vi "mlink_scan_trigger_encoder.vi"(6 "module":u8, 7 "trigger type":T1, 8 "error in (no error)":errorcluster, 9 "slope":u8, 10 "position":i32, 11 "connection ID":i32=-1) -> (0 "error out":errorcluster, 3 "connection ID out":i32)   [LabVIEW 2009, in "MicroDAQ.lvlib" / "mlink.lvlib"]
doc: "This function configures Encoder value trigger for AO/AI scan operation. The function shall \nbe called after scan initialization function. The trigger argument determines if function affects \nAO or AI trigger settings. The module argument determines which encoder module position \nvalue will be used. The slope argument defines if trigger shall occur for value greater or lower \nthen position argument."
uses:
  <instrlib>/MicroDAQ/Mlink library wraper/mlink.lvlib
  <instrlib>/MicroDAQ/Tools/Trigger type.ctl
  <instrlib>/MicroDAQ/MLink32.dll
  <instrlib>/MicroDAQ/MicroDAQ.lvlib
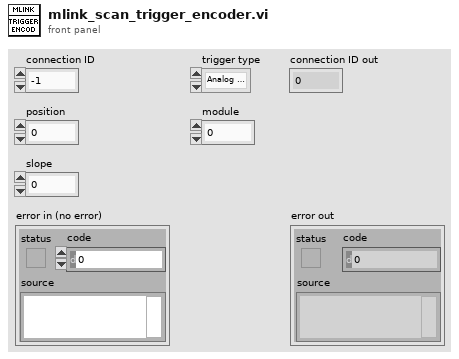
[diagram p1: front panel]
types:
  T1 = typedef "MicroDAQ.lvlib/Trigger type.ctl" = enum8{"Analog output", "Analog input"}
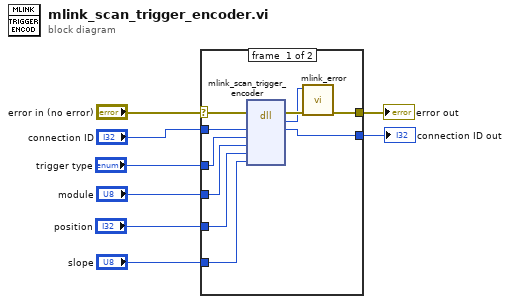
[diagram p0: block diagram]
diagram:
  n1 = case shown="No Error" "error in (no error)" {
    selector: "error in (no error)" -> [w18 w20]
    tunnel: "connection ID" -> [w17 w19]
    tunnel: [w16 w19] -> w6
    tunnel: [w13 w20] -> w5
    tunnel: "trigger type" -> [w12 _]
    tunnel: "module" -> [w11 _]
    tunnel: "position" -> [w10 _]
    tunnel: "slope" -> [w9 _]
    frame #0 {
      n2 = dll-call lib="C:/Program Files (x86)/National Instruments/LabVIEW 2009/instr.lib/MicroDAQ/MLink32.dll" fn="mlink_scan_trigger_encoder" ("MLink64.dll:mlink_dsp_run")(error in=w18, "link_fd"=w17, "trigger"=w12, "module"=w11, "position"=w10, "slope"=w9) -> (error out=w15:errorcluster, "return type"=w14:i32, "link_fd"=w16:i32)  [unwired: 6 in, 1 out]
      n3 = call <instrlib>:"mlink_error.vi"("error in (no error)"=w15, "error code"=w14) -> ("error out"=w13:errorcluster)  [unwired: 9 in]
    }
    frame #1 {
    }
  }
  "connection ID out" <- w6
  "error out" <- w5
